vi "Write Handle Mouse Down Msg.vi"(6 "Handle Mouse Down Msg":refnum<class "Handle Mouse Down Msg.lvclass">, 11 "Test Executive Builder Event Filter in":refnum<class "Test Executive Builder Event Filter.lvclass">) -> (3 "Test Executive Builder Event Filter out":refnum<class "Test Executive Builder Event Filter.lvclass">)   [LabVIEW 2017, in "Test Executive Builder Event Filter.lvclass"]
uses:
  <vilib>/gpm_packages/@cs/Test-executive-builder/Source/Test Executive Builder View/Test Executive Builer Event Filter/Test Executive Builder Event Filter.lvclass
  <vilib>/gpm_packages/@cs/Test-executive-builder/Source/Test Executive Builder View/Test Executive Builder View Messages/Handle Mouse Down Msg/Handle Mouse Down Msg.lvclass
  <vilib>/gpm_packages/@cs/Test-executive-builder/Source/Test Executive Builder View/Test Executive Builer Event Filter/Test Executive Builder Event Filter.lvclass/Test Executive Builder Event Filter.ctl
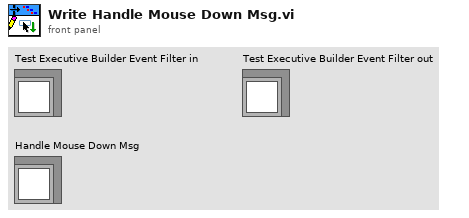
[diagram p1: front panel]
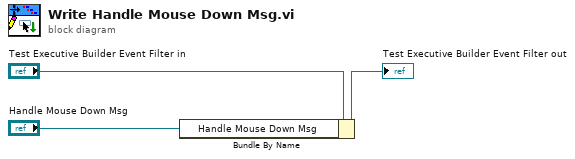
[diagram p0: block diagram]
diagram:
  n1 = Bundle By Name(cluster="Test Executive Builder Event Filter in", "Handle Mouse Down Msg"="Handle Mouse Down Msg") -> (→"Test Executive Builder Event Filter out":refnum<class "Test Executive Builder Event Filter.lvclass">)
